vi "Config-Stress-Parameters.vi"(0 "VISA session":refnum<visa-resource-name>, 1 "pulse count (0: free run)":i32, 5 "stress mode":bool, 7 "stop condition (continue:0)\n(set to 0 when duration <=10 sec)":u8(ring) items=["always continue", "stop at any abnormal", "stop at compliance"], 9 "filter state":bool, 11 "error in (no error)":errorcluster, 12 "duration (0: free run)":dbl format="%.4f", 13 "hold time (sec)":dbl format="%^.4e") -> (4 "VISA resource name out":refnum<visa-resource-name>, 15 "error out":errorcluster)   [LabVIEW 2016, in "Agilent 415X Series.lvlib"]
doc: "This VI configures the stress parameters (duration, hold time, filter, stress stop condition and etc.) Constant sources are configured by HP415xA Config Stress Channel.vi.\n\nThis VI does NOT perform any error checking. For example, it does not verify the existence of a PGU and its mode (SYNC or NonSYNC) before sending the pulse count."
uses:
  Agilent 415X Series.lvlib
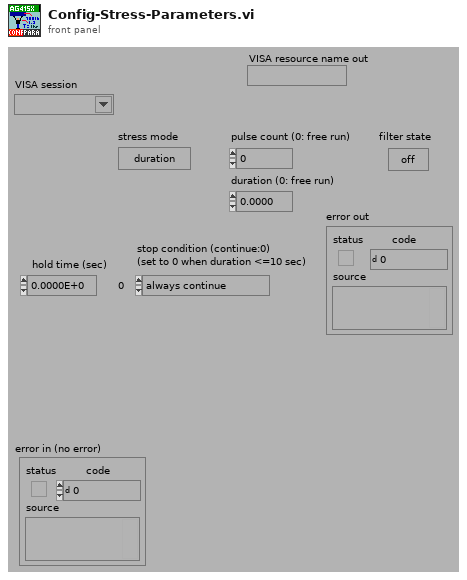
[diagram p1: front panel]
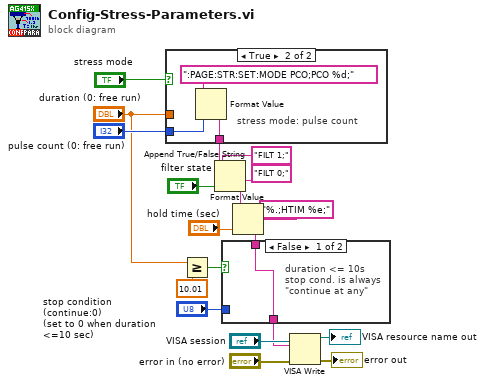
[diagram p0: block diagram]
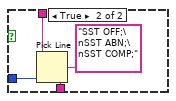
[diagram p2: hidden frame]
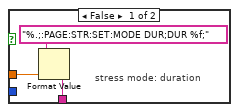
[diagram p3: hidden frame]
diagram:
  n1 = case shown="True" "stress mode" {
    tunnel: "duration (0: free run)" -> [w22 _]
    tunnel: "pulse count (0: free run)" -> [_ w24]
    tunnel: [w20 w23] -> w14
    frame False {
      # "stress mode: duration"
      n2 = Format Value(format string="%.;:PAGE:STR:SET:MODE DUR;DUR %f;", value (0)=w22) -> (output string=w20:string)  [unwired: 1 in]
    }
    frame True {
      # "stress mode: pulse count"
      n3 = Format Value(format string=":PAGE:STR:SET:MODE PCO;PCO %d;", value (0)=w24) -> (output string=w23:string)  [unwired: 1 in]
    }
  }
  n4 = Greater Or Equal?(x="duration (0: free run)", y=10.01) -> (x >= y?=w7:bool)
  n5 = Append True/False String(1:"filter state", 2:"FILT 0;", 3:"FILT 1;", 4:w14) -> (0:w2:string)
  n6 = Format Value(string ("")=w2, format string="%.;HTIM %e;", value (0)="hold time (sec)") -> (output string=w8:string)
  n7 = case shown="False" w7 {
    tunnel: "stop condition (continue:0)\n(set to 0 when duration <=10 sec)" -> [_ w30]
    tunnel: w8 -> [w26 w29]
    tunnel: [w26 w27] -> w3
    frame False {
      # "duration <= 10s\nstop cond. is always\n\"continue at any\""
    }
    frame True {
      n8 = Pick Line(string ("")=w29, multi-line string="SST OFF;\nSST ABN;\nSST COMP;", line index=w30) -> (output string=w27:string)
    }
  }
  n9 = VISA Write(VISA resource name="VISA session", write buffer=w3, error in (no error)="error in (no error)") -> (VISA resource name out=→"VISA resource name out":refnum<visa-resource-name>, error out=→"error out":errorcluster)  [unwired: 1 out]
